vi "FGV_EstadoMotores.vi"(7 "Control":T3, 8 "error in (no error)":errorcluster, 9 "edoMotores3_in":u8, 10 "edoMotores2_in":u8, 11 "edoMotores_in":u8) -> (0 "error out":errorcluster, 2 "Estados":T2, 3 "Estados":bool)   [LabVIEW 2026]
uses:
  Ctrl_EstadosMotor.ctl
  Ctrl_EstadoMotorEsp.ctl
  Cluster_EstadoMotores.ctl
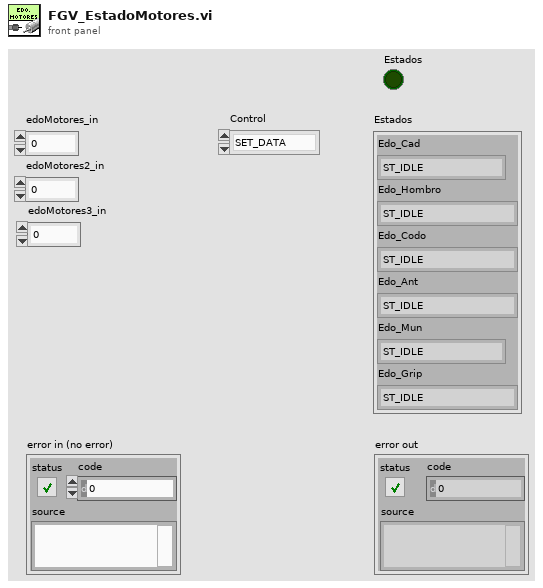
[diagram p1: front panel]
types:
  T1 = typedef "Ctrl_EstadoMotorEsp.ctl" = enum16{"ST_IDLE", "ST_MOVIENDO", "ST_HOMING", "ST_ERROR_TRABADO"}
  T2 = cluster{"Edo_Cad":T1, "Edo_Hombro":T1, "Edo_Codo":T1, "Edo_Ant":T1, "Edo_Mun":T1, "Edo_Grip":T1}
  T3 = typedef "Ctrl_EstadosMotor.ctl" = enum16{"SET_DATA", "GET_DATA", "START"}
  T4 = typedef "Cluster_EstadoMotores.ctl" = cluster{"Edo_Cad":T1, "Edo_Hombro":T1, "Edo_Codo":T1, "Edo_Ant":T1, "Edo_Mun":T1, "Edo_Grip":T1}
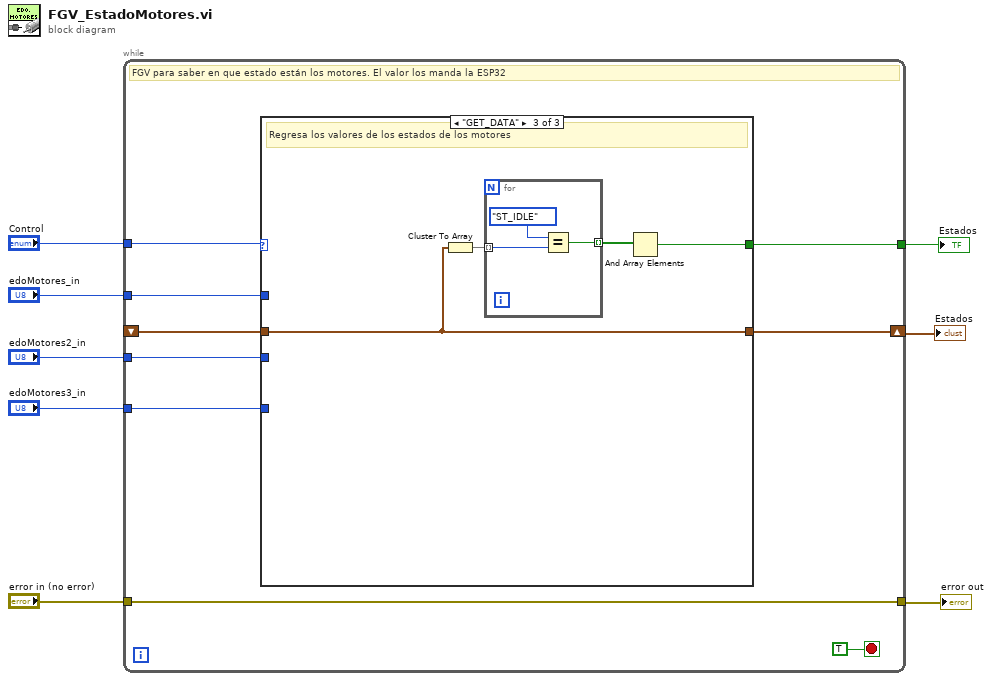
[diagram p0: block diagram]
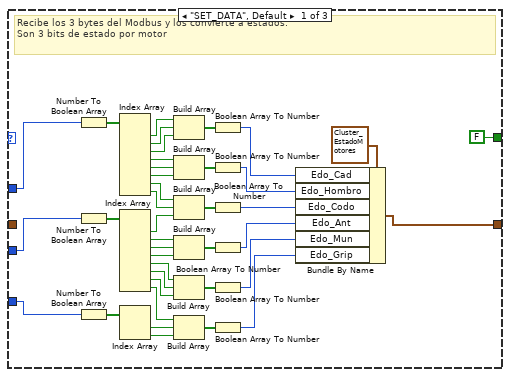
[diagram p2: hidden frame]
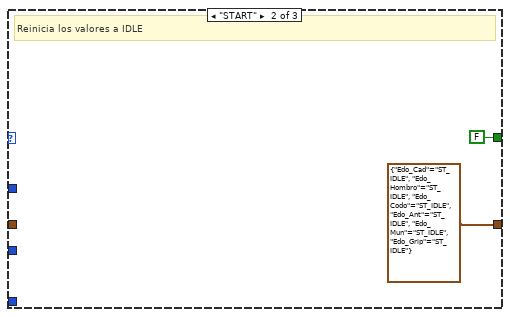
[diagram p3: hidden frame]
diagram:
  n1 = while {
    tunnel: "error in (no error)" -> [w17]
    tunnel: [w17] -> w7
    tunnel: "Control" -> [w15]
    tunnel: "edoMotores_in" -> [w14]
    tunnel: "edoMotores2_in" -> [w13]
    tunnel: "edoMotores3_in" -> [w12]
    shift-right: [w11] -> w2
    shift-left: _ -> [w10]
    tunnel: [w9] -> w1
    stop <- TRUE stop-if-true
    # "FGV para saber en que estado están los motores. El valor los manda la ESP32"
    n2 = case shown="\"GET_DATA\"" w15 {
      tunnel: w14 -> [w55 _ _]
      tunnel: w13 -> [w38 _ _]
      tunnel: w12 -> [w22 _ _]
      tunnel: [w53 T2 {"Edo_Cad"=enum."ST_IDLE", "Edo_Hombro"=enum."ST_IDLE", "Edo_Codo"=enum."ST_IDLE", "Edo_Ant"=enum."ST_IDLE", "Edo_Mun"=enum."ST_IDLE", "Edo_Grip"=enum."ST_IDLE"} w62] -> w11
      tunnel: w10 -> [_ _ w62]
      tunnel: [FALSE FALSE w59] -> w9
      frame "SET_DATA", Default {
        # "Recibe los 3 bytes del Modbus y los convierte a estados.\nSon 3 bits de estado por motor"
        n3 = Number To Boolean Array(number=w55) -> (Boolean array=w54:bool[])
        n4 = Number To Boolean Array(number=w38) -> (Boolean array=w37:bool[])
        n5 = Number To Boolean Array(number=w22) -> (Boolean array=w21:bool[])
        n6 = Index Array(array=w54) -> (element #1=w52:bool, element #2=w51:bool, element #3=w50:bool, element #4=w47:bool, element #5=w46:bool, element #6=w45:bool, element #7=w42:bool, element #8=w41:bool)  [unwired: 8 in]
        n7 = Index Array(array=w37) -> (element #1=w36:bool, element #2=w35:bool, element #3=w34:bool, element #4=w33:bool, element #5=w32:bool, element #6=w31:bool, element #7=w30:bool, element #8=w29:bool)  [unwired: 8 in]
        n8 = Index Array(array=w21) -> (element #1=w20:bool, element #2=w19:bool)  [unwired: 2 in]
        n9 = Build Array(w52, w51, w50) -> (w49:bool[])
        n10 = Build Array(w47, w46, w45) -> (w43:bool[])
        n11 = Build Array(w42, w41, w36) -> (w39:bool[])
        n12 = Build Array(w35, w34, w33) -> (w28:bool[])
        n13 = Build Array(w32, w31, w30) -> (w27:bool[])
        n14 = Build Array(w29, w20, w19) -> (w26:bool[])
        n15 = Boolean Array To Number(Boolean array=w49) -> (number=w48:u32)
        n16 = Boolean Array To Number(Boolean array=w43) -> (number=w44:u32)
        n17 = Boolean Array To Number(Boolean array=w39) -> (number=w40:u32)
        n18 = Boolean Array To Number(Boolean array=w28) -> (number=w23:u32)
        n19 = Boolean Array To Number(Boolean array=w27) -> (number=w24:u32)
        n20 = Boolean Array To Number(Boolean array=w26) -> (number=w25:u32)
        n21 = Bundle By Name(cluster=T4 {"Edo_Cad"=enum."ST_IDLE", "Edo_Hombro"=enum."ST_IDLE", "Edo_Codo"=enum."ST_IDLE", "Edo_Ant"=enum."ST_IDLE", "Edo_Mun"=enum."ST_IDLE", "Edo_Grip"=enum."ST_IDLE"}, "Edo_Cad"=w48, "Edo_Hombro"=w44, "Edo_Codo"=w40, "Edo_Ant"=w23, "Edo_Mun"=w24, "Edo_Grip"=w25) -> (w53:T4)
      }
      frame "START" {
        # "Reinicia los valores a IDLE"
      }
      frame "GET_DATA" {
        # "Regresa los valores de los estados de los motores"
        n22 = Cluster To Array(cluster=w62) -> (array=w61:T1[])
        n23 = for {
          tunnel: w61 -> [w65] mode=indexing
          tunnel: [w63] -> w60 mode=indexing
          n24 = Equal?(x=Ctrl_EstadoMotorEsp."ST_IDLE", y=w65) -> (x = y?=w63:bool)
        }
        n25 = And Array Elements(Boolean array=w60) -> (logical AND=w59:bool)
      }
    }
  }
  "error out" <- w7
  "Estados" <- w2
  "Estados" <- w1
